vi "NIMS_DF_DefaultCast_iir_comb.vi"(10 "Number of Outputs Requested":i32, 11 "Input Types":refnum<class "NDArray.lvclass">[](array[class])) -> (0 "Error Enum":T2, 3 "Algorithm VI Path":path, 5 "Output Vector Orientations (all row)":T1[](array[typedef]))   [LabVIEW 2017, in "NI_DigFilter_MathScript.lvlib"]
uses:
  <vilib>/addons/Digital Filter Design/NI_DigFilter_MathScript.lvlib
  <vilib>/imath/engines/lvmath2/MathScriptCompiler/Type/NDArray.llb/NDArray.lvclass
  <vilib>/imath/engines/lvmath/Functions/Error Handling/error.ctl
  <vilib>/imath/engines/lvmath2/MathScriptCompiler/BuiltInFunctionSupport/BuiltInFunctionSupport.llb/VectorOrientation.ctl
  <vilib>/imath/engines/lvmath2/MathScriptCompiler/BuiltInFunctionSupport/BuiltInFunctionSupport.llb/BuiltInFunctionSupport.lvlib
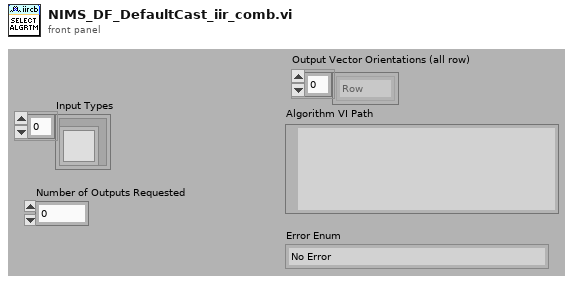
[diagram p1: front panel]
types:
  T1 = typedef "BuiltInFunctionSupport.lvlib/VectorOrientation.ctl" = enum16{"Row", "Column"}
  T2 = typedef "error.ctl" = enum16{"No Error", "Problem", "Input type must not be void", "Incorrect number of parameters", "Function not defined for non-numeric types", "An output variable of the user-defined function is undefined", "Function only defined for character arrays", "Function not defined for boolean, character, or single precision", "Function not defined for complex types", "Not a valid operation", "Inputs must be scalar", "Input matrices are not the same size", "Function only available on RT", "Input matrices must be nonnegative integers of the same type", "Arguments must be non-negative integers less than bitmax", "Number to complement must be less than 2^N", "Bit to get is outside range", "Bit to set is outside range", "Input must be real type ", "At least one parameter must be scalar", "Unable to display plug-in data on RT", "Function not defined for higher dimensional matrices", "Invalid attributes", "Wrong Type of Input Arguments", "Wrong Argument Option", "Invalid file identifier", "Indices must be real positive integers", "The variable is not a matrix data type.", "Number of elements must be the same for indices and values", "You cannot replace elements of a matrix with non-matrix data types.", "Cannot resize a 2D matrix with a linear index", "Unknown variable or symbol", "Indices out of range", "Empty matrix deletion can not be used with two indices", "Number of rows and columns must be the same for indices and values.", "Complex cannot be converted to Boolean", "Char cannot be converted to Boolean", "int64 cannot be converted to Boolean", "uint64 cannot be converted to Boolean", "You cannot convert a Boolean to a character.", "Incompatible input size in 3D surface function", "All rows must have the same number of columns", "Incompatible types", "Invalid matrix dimensions", "Dimension must be 1 or 2", "Base must be an integer between 2 and 36", "Invalid input", "Square matrix required", "Function 'timerstart' must be called before 'timerstop'", "Arguments must be positive real", "Step must not be zero", "Wrong number of input arguments", "Wrong number of output arguments", "Too many index arguments", "Input scalar must be >= 0", "Input scalar must be positive", "Input scalar must not be 0", "Input scalar must be in range [0,1]", "Can't use conditionally defined variable that's undefined", "Input must be a vector", "RT Exec Trace Toolkit not licensed", "Empty vector error", "All elements must be in domain [-1,1]", "All real elements of input vector must be >= 0", "All elements of input vector must be positive", "Values of input vectors are not compatible", "DAQmx not installed", "Input vector must be an increasing vector", "Dereferenced field does not exist within the struct", "A vector or matrix of structures must be indexed before it can be dereferenced", "Lenths of two input vectors are not compatible", "Invalid fieldname", "Empty matrix error", "Cannot use '.' on a type other than Struct", "Unused074", "Data type of the struct's field name is invalid", "Using . to dereference data that is not a struct", "Input struct contains invalid type ", "Size of input matrix is incompatible with input size", "Invalid format specifier", "Could not find field within struct", "Bad permutation array", "Mismatched fieldnames", "ode: User Function could not be opened", "ode: User Function signature does not meet ode requirements", "Unused085", "RunTime: MathScript could not be compiled", "Unknown function", "Only scalars and strings supported", "ode: User Function signature has incorrect number of inputs", "ode:User Function signature has incorrect number of outputs", "Range is too large", "End used without variable", "Function not available (RTE)", "Custom user error", "Arguments must be integers less than bitmax", "Shared library not found", "Header file not found", "Shared library already loaded", "Shared library not loaded", "Shared library function not found", "Shared library string return problem", "Problem calling shared library function", "Problem loading shared library from OS", "Problem parsing shared library header file", "Shared library incompatible types", "Shared library unsupported return type", "Shared library function not exported", "Shared library unsupported input type", "Problem unloading shared library from OS", "Function only available from UI", "Function specified in argument is missing", "An internal error has occurred", "Invalid object", "Invalid property", "Read-only property", "A break command has occurred", "A continue command has occurred", "A return command has occurred", "ode: times parameter invalid", "Function specified in argument has incorrect signature", "Function not found in file", "Reserved keyword cannot be defined as variable", "Reserved keyword cannot be defined as a function or script", "Arguments must be string literals", "Function not supported on this platform", "All columns must have the same number of rows", "Function ignored in RTE warning", "Cannot use : as a parameter that is not a variable", "Output can't be coerced to requested type", "Function not supported on current target", "Variable dependent on an unwired function input", "Unused132", "Unused133", "Unused134", "Unused135", "Unused136", "Unused137", "Unused138", "Unused139", "Global/Persistent must only take constants as arguments.", "Varargin must be last input in the function definition.", "Varargout must be last output in the function definition.", "Invalid output type. Cannot output a cell array of any type other than string.", "Invalid output type. Type is a dynamic struct.", "Invalid output type. Type is a struct that has a field whose type is not known until run-time", "Invalid output type. Type is a struct that has a field which is a plot object.", "MathScript parser DLL missing", "MathScript requires LabVIEW Full", "MathScript license is invalid or missing", "Varargout not supported except in assignments."}
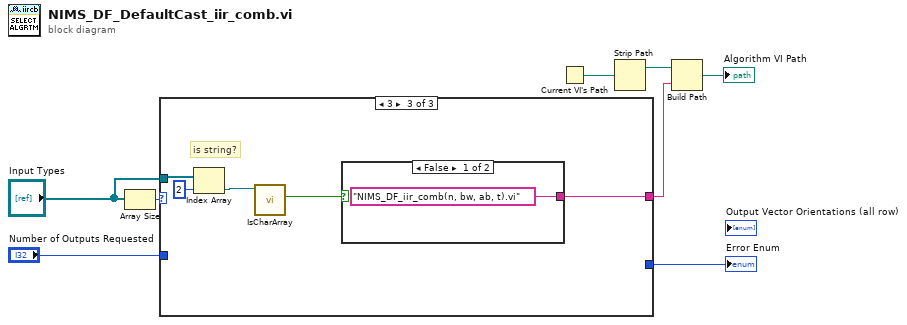
[diagram p0: block diagram]
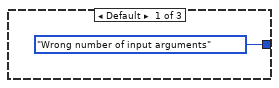
[diagram p2: hidden frame]
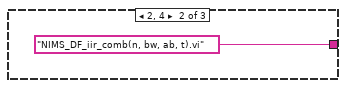
[diagram p3: hidden frame]
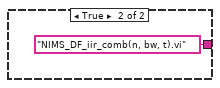
[diagram p4: hidden frame]
diagram:
  n1 = Array Size(array="Input Types") -> (size(s)=w8:i32)
  n2 = case shown="3" w8 {
    tunnel: "Input Types" -> [_ _ w14]
    tunnel: [error."Wrong number of input arguments" ("Error Enum") _ _] -> w4
    tunnel: [_ "NIMS_DF_iir_comb(n, bw, ab, t).vi" ("name or relative path") w15] -> w3
    tunnel: "Number of Outputs Requested" -> [_ _ _]
    frame Default {
    }
    frame 2, 4 {
    }
    frame 3 {
      # "is string?"
      n3 = Index Array(array=w14, index=2) -> (element=w13:refnum<class "NDArray.lvclass">)
      n4 = call-dynamic "IsCharArray.vi"("NDArray in"=w13) -> ("Is Char PlugIn?"=w12:bool)  [unwired: 10 out]
      n5 = case shown="False" w12 {
        tunnel: ["NIMS_DF_iir_comb(n, bw, ab, t).vi" ("name or relative path") "NIMS_DF_iir_comb(n, bw, t).vi" ("name or relative path")] -> w15
        frame False {
        }
        frame True {
        }
      }
    }
  }
  "Error Enum" <- w4
  n6 = Current VI's Path() -> (path=w7:path)
  n7 = Strip Path(path=w7) -> (stripped path=w5:path)  [unwired: 1 out]
  n8 = Build Path(base path=w5, name or relative path=w3) -> (appended path=→"Algorithm VI Path":path)
